vi "dfd_Convert ZPK to String.vi"(5 "indent order":i32, 6 "type (FLP)":enum16{"FLP", "FXP"}(ring), 7 "format string":string="%-+024.16e", 11 "filter":T1={"mSRate_Fs"=1.0, "mSRate_Version"="1.0", "mSRate_Comments"="", "mSRate_OrgCoef"={"type"=enum."Undefined", "gain"=1.0, "coef a (k)"=[], "coef b (v)"=[]}, "mSRate_CurCoef"={"type"=enum."Undefined", "gain"=1.0, "coef a (k)"=[], "coef b (v)"=[]}, "mSRate_Quantized?"=FALSE, "mSRate_QCoef"={"type"=enum."Undefined", "gain"=1.0, "coef a (k)"=[], "coef b (v)"=[]}, "mSRate_QSettings"=[], "mSRate_Order"=0, "mSRate_Scaling"={"mSRate_ScaleByPowerOf2?"=FALSE, "mSRate_ScaleType"=enum."No Norm"}} {"mSRate_QSettings"."source" items=["Coef a/k"=0, "Coef b/v"=7, "Input"=1, "Output"=2, "Multiplicand"=3, "Product"=4, "Sum"=5, "Delay"=6, "Gain"=8]}) -> (3 "xml string":string)   [LabVIEW 2017, in "NI_DigFilter_Process.lvlib"]
uses:
  <vilib>/addons/Digital Filter Design/NI_DigFilter_Process.lvlib
  <vilib>/addons/Digital Filter Design/_Objects.llb/DFD Filter Obj.ctl
  <vilib>/addons/Digital Filter Design/_Objects.llb/DFD Filter Coef.ctl
  <vilib>/addons/Digital Filter Design/_Objects.llb/DFD Filter Structure Type Selector.ctl
  <vilib>/addons/Digital Filter Design/_Objects.llb/dfd_Internal Quantization Settings.ctl
  <vilib>/addons/Digital Filter Design/_Objects.llb/dfd_Internal Quantization Srcs.ctl
  <vilib>/addons/Digital Filter Design/_Objects.llb/DFD Coef Norm Type.ctl
  <vilib>/addons/Digital Filter Design/NI_DigFilterLicensed.lvlib
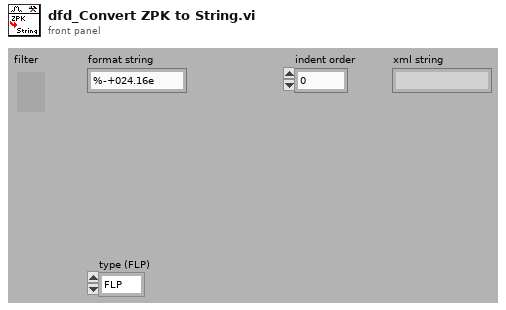
[diagram p1: front panel]
types:
  T1 = typedef "NI_DigFilterLicensed.lvlib/DFD Filter Obj.ctl" = cluster{"mSRate_Fs":dbl, "mSRate_Version":string, "mSRate_Comments":string, "mSRate_OrgCoef":T2, "mSRate_CurCoef":T2, "mSRate_Quantized?":bool, "mSRate_QCoef":T2, "mSRate_QSettings":T4[], "mSRate_Order":i32, "mSRate_Scaling":cluster{"mSRate_ScaleByPowerOf2?":bool, "mSRate_ScaleType":T6}}
  T2 = typedef "NI_DigFilterLicensed.lvlib/DFD Filter Coef.ctl" = cluster{"type":T3, "gain":dbl, "coef a (k)":dbl[], "coef b (v)":dbl[]}
  T3 = typedef "NI_DigFilterLicensed.lvlib/DFD Filter Structure Type Selector.ctl" = enum16{"Undefined", "FIR Direct Form", "FIR Direct Form Transposed", "FIR Symmetric", "FIR Antisymmetric", "IIR Direct Form I", "IIR Direct Form I Transposed", "IIR Direct Form II", "IIR Direct Form II Transposed", "IIR Cascaded Second Order Sections Form I", "IIR Cascaded Second Order Sections Form I Transposed", "IIR Cascaded Second Order Sections Form II", "IIR Cascaded Second Order Sections Form II Transposed", "Lattice Allpass (basic sections)", "Lattice Allpass (one multiplier sections)", "Lattice Allpass (normalized sections)", "Lattice AR (basic sections)", "Lattice AR (one multiplier sections)", "Lattice AR (normalized sections)", "Lattice MA (minimum phase)", "Lattice MA (maximum phase)", "Lattice ARMA (basic sections)", "Lattice ARMA (one multiplier sections)", "Lattice ARMA (normalized sections)"}
  T4 = typedef "NI_DigFilterLicensed.lvlib/dfd_Internal Quantization Settings.ctl" = cluster{"source":T5, "wl":i16, "iwl":i16, "overflow mode":enum16{"Saturation", "Wrap"}, "rounding mode":enum16{"Nearest", "Truncation"}, "signed?":bool}
  T5 = typedef "NI_DigFilterLicensed.lvlib/dfd_Internal Quantization Srcs.ctl" = u16
  T6 = typedef "NI_DigFilterLicensed.lvlib/DFD Coef Norm Type.ctl" = enum16{"No Norm", "Time Domain 1-Norm", "Time Domain 2-Norm", "Time Domain Inf-Norm"}
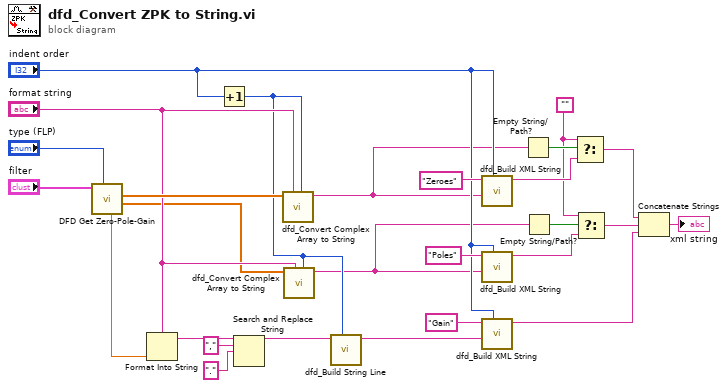
[diagram p0: block diagram]
diagram:
  w5 = ""
  n1 = call <vilib>:"DFD Get Zero-Pole-Gain.vi"("type (FLP)"="type (FLP)", "filter in"="filter") -> ("poles"=w15:cdb[], "zeroes"=w18:cdb[], "gain"=w14:dbl)  [unwired: 1 in, 6 out]
  n2 = Format Into String(format string="format string", w14) -> (resulting string=w2:string)  [unwired: 2 in, 1 out]
  n3 = Increment(x="indent order") -> (x+1=w16:i32)
  n4 = Search and Replace String(input string=w2, search string=",", replace string="." ("replace string (\"\")")) -> (result string=w1:string)  [unwired: 2 in, 6 out]
  n5 = call <vilib>:"dfd_Convert Complex Array to String.vi"("indent order"=w16, "format string"="format string", "roots"=w18) -> ("string"=w12:string)  [unwired: 1 in, 7 out]
  n6 = call <vilib>:"dfd_Convert Complex Array to String.vi"("indent order"=w16, "format string"="format string", "roots"=w15) -> ("string"=w10:string)  [unwired: 1 in, 7 out]
  n7 = call <vilib>:"dfd_Build String Line.vi"("indent order"=w16, "string"=w1) -> ("string line"=w20:string)  [unwired: 9 out]
  n8 = call <vilib>:"dfd_Build XML String.vi"("indent order"="indent order", "string in"=w12, "element name"="Zeroes") -> ("xml string out"=w8:string)  [unwired: 1 in, 7 out]
  n9 = call <vilib>:"dfd_Build XML String.vi"("indent order"="indent order", "string in"=w10, "element name"="Poles") -> ("xml string out"=w7:string)  [unwired: 1 in, 7 out]
  n10 = call <vilib>:"dfd_Build XML String.vi"("indent order"="indent order", "string in"=w20, "element name"="Gain") -> ("xml string out"=w24:string)  [unwired: 1 in, 7 out]
  n11 = Empty String/Path?(string/path=w12) -> (empty?=w13:bool)
  n12 = Empty String/Path?(string/path=w10) -> (empty?=w11:bool)
  n13 = Select(t=w5, s=w13, f=w8) -> (s? t:f=w9:string)
  n14 = Select(t=w5, s=w11, f=w7) -> (s? t:f=w6:string)
  n15 = Concatenate Strings(w9, w6, w24) -> (→"xml string":string)
